vi "Bool_VIG.vi"(6 "Set(t) Reset(f) \nDominant":bool, 7 "First call":bool, 8 "Latch(t) Edge(f)":bool, 9 "Initial State":bool, 10 "Reset":bool, 11 "Input/Set":bool) -> (0 "Change":bool, 1 "Fall":bool, 2 "Rise":bool, 3 "Output":bool)   [LabVIEW 2020]
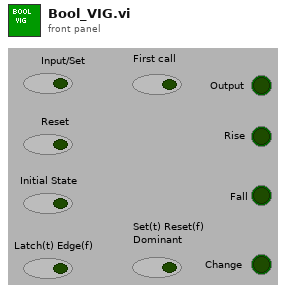
[diagram p1: front panel]
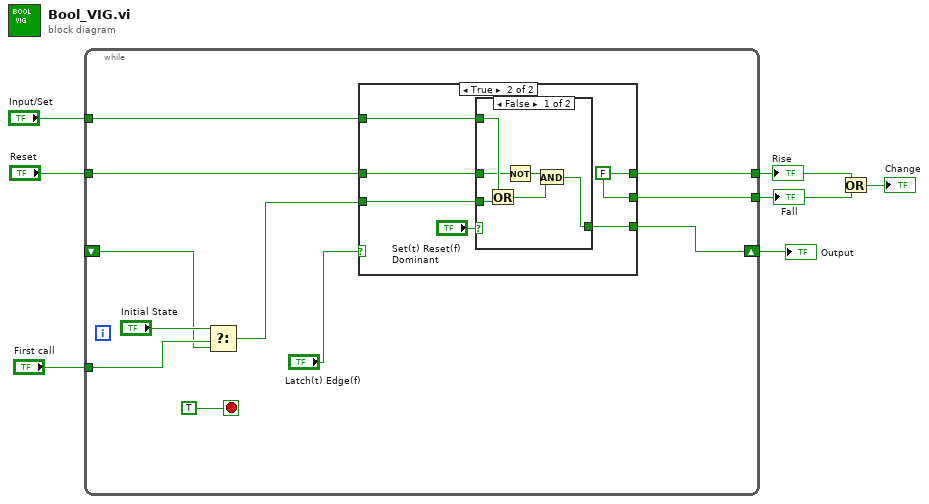
[diagram p0: block diagram]
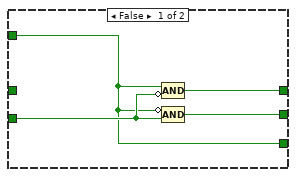
[diagram p2: hidden frame]
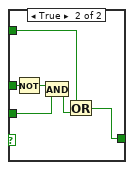
[diagram p3: hidden frame]
diagram:
  n1 = while {
    tunnel: "Reset" -> [w16]
    tunnel: [w17] -> w5
    tunnel: [w18] -> w6
    tunnel: "First call" -> [w11]
    tunnel: "Input/Set" -> [w15]
    shift-right: [w14] -> w1
    shift-left: _ -> [w9]
    stop <- TRUE stop-if-true
    n2 = Select(t="Initial State", s=w11, f=w9) -> (s? t:f=w8:bool)
    n3 = case shown="True" "Latch(t) Edge(f)" {
      tunnel: w8 -> [w22 w27]
      tunnel: [w21 w25] -> w18
      tunnel: [w20 w25] -> w17
      tunnel: w15 -> [w19 w28]
      tunnel: [w19 w26] -> w14
      tunnel: w16 -> [_ w24]
      frame False {
        n4 = Compound Arithmetic op=AND(w19, invert w22) -> (w21:bool)
        n5 = Compound Arithmetic op=AND(invert w19, w22) -> (w20:bool)
      }
      frame True {
        w25 = FALSE
        n6 = case shown="False" "Set(t) Reset(f) \nDominant" {
          tunnel: w28 -> [w34 w35]
          tunnel: w27 -> [w33 w37]
          tunnel: [w32 w38] -> w26
          tunnel: w24 -> [w30 w39]
          frame False {
            n7 = Or(x=w34, y=w33) -> (x .or. y?=w31:bool)
            n8 = Not(x=w30) -> (.not. x?=w29:bool)
            n9 = And(x=w29, y=w31) -> (x .and. y?=w32:bool)
          }
          frame True {
            n10 = Not(x=w39) -> (.not. x?=w40:bool)
            n11 = And(x=w40, y=w37) -> (x .and. y?=w36:bool)
            n12 = Or(x=w35, y=w36) -> (x .or. y?=w38:bool)
          }
        }
      }
    }
  }
  "Rise" <- w6
  "Fall" <- w5
  "Output" <- w1
  n13 = Or(x=w6, y=w5) -> (x .or. y?=→"Change":bool)
